vi "PH_DeformableMirror.evt call SetChannel.vi"(0 "i ref in":refnum<vi>, 1 "Object":string="N/A", 3 "channel":u32, 4 "voltage":dbl, 5 "error in (no error)":errorcluster, 7 "Hysteresis Compensation? (false)":bool) -> (14 "i ref out":refnum<vi>, 19 "error out":errorcluster)   [LabVIEW 2014, in "PH_DeformableMirror.lvlib"]
uses:
  PH_DeformableMirror.lvlib
  CSCore/CSSystem/CoreLib/CoreLib.int 2 byte array.vi
  CSCore/CSSystem/CoreLib/CoreLib.double 2 byte array.vi
  CSCore/CSSystem/CoreLib/CoreLib.short 2 byte array.vi
  CSCore/CSSystem/CoreLib/CoreLib.lvlib
  CSCore/BaseProcess/BaseProcess.lvlib
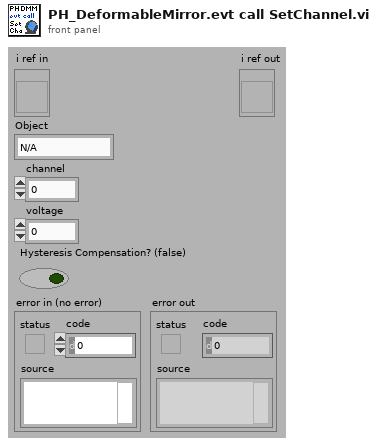
[diagram p1: front panel]
types:
  T1 = typedef "CoreDefs.rawDataType.ctl" = i8[]
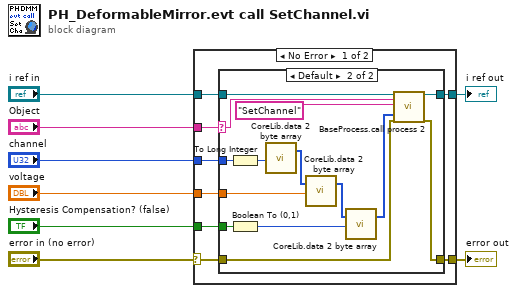
[diagram p0: block diagram]
diagram:
  n1 = case shown="No Error" "error in (no error)" {
    selector: "error in (no error)" -> [w13 w33]
    tunnel: "i ref in" -> [w16 w34]
    tunnel: [w15 w34] -> w7
    tunnel: [w14 w33] -> w6
    tunnel: "Object" -> [w12 _]
    tunnel: "voltage" -> [w11 _]
    tunnel: "channel" -> [w10 _]
    tunnel: "Hysteresis Compensation? (false)" -> [w9 _]
    frame No Error {
      n2 = case shown="Default" w12 {
        selector: w12 -> [_ w28]
        tunnel: w16 -> [w18 w32]
        tunnel: [w18 w31] -> w15
        tunnel: [w17 w30] -> w14
        tunnel: w13 -> [w17 w29]
        tunnel: w11 -> [_ w24]
        tunnel: w10 -> [_ w25]
        tunnel: w9 -> [_ w22]
        frame "", "N/A" {
        }
        frame Default {
          n3 = To Long Integer(number=w25) -> (32bit integer=w23:i32)
          n4 = Boolean To (0,1)(Boolean=w22) -> (0, 1=w21:i16)
          n5 = call-poly "CoreLib.data 2 byte array.vi"("i32"=w23) -> ("byteArray out"=w26:T1)  [unwired: 18 in]
          n6 = call-poly "CoreLib.data 2 byte array.vi"("byteArray"=w26, "f64"=w24) -> ("byteArray out"=w20:T1)  [unwired: 17 in]
          n7 = call-poly "CoreLib.data 2 byte array.vi"("byteArray"=w20, "i16"=w21) -> ("byteArray out"=w19:T1)  [unwired: 17 in]
          n8 = call "BaseProcess.call process 2.vi"("i ref in"=w32, "Object"=w28, "Selector"="SetChannel", "Data"=w19, "error in (no error)"=w29) -> ("i ref out"=w31:refnum<vi>, "error out"=w30:errorcluster)  [unwired: 13 in]
        }
      }
    }
    frame Error {
    }
  }
  "error out" <- w6
  "i ref out" <- w7
